vi "Close.vi"(7 "Micropulse # In":i32, 8 "error in (no error)":errorcluster) -> (0 "error out":errorcluster, 5 "Micropulse # Out":i32)   [LabVIEW 2026, in "MicroPulse_Driver.lvlib"]
doc: "Performs an instrument error query before terminating the software connection to the instrument."
uses:
  MicroPulse_Driver.lvlib
  Private/MP-Registry Action-Enum.ctl
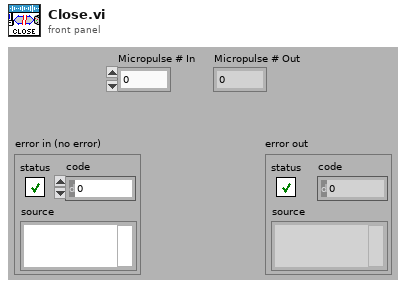
[diagram p1: front panel]
types:
  T1 = typedef "MicroPulse_Driver.lvlib/MP-Registry Action-Enum.ctl" = enum16{"Read", "Add Test", "Add Command", "Add Gate Command", "Add Encoder Command", "Clear Command  List", "Set Registry", "Set System Details", "Set DOF", "Set Velocity", "Disable Asynch Reads", "Enable Asynch Reads", "Add Connection", "Disconnect", "Shutdown"}
  T2 = typedef "MicroPulse_Driver.lvlib/TCP config.ctl" = cluster{"Connection ID":refnum<k5>, "IP address":string, "host port":u16, "OC timeout":i32, "Read timeout":i32, "Write timeout":i32}
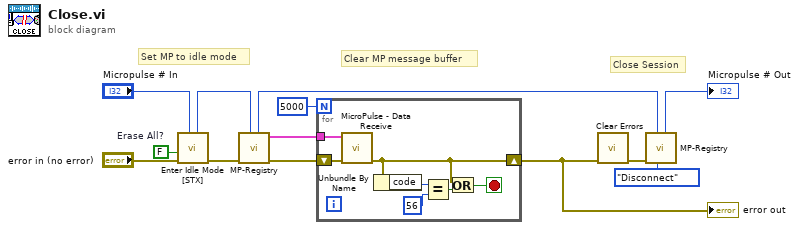
[diagram p0: block diagram]
diagram:
  w10 = FALSE  # Erase All?
  # "Set MP to idle mode"
  # "Clear MP message buffer"
  # "Close Session"
  n1 = call "Enter Idle Mode [STX].vi"("Micropulse # In"="Micropulse # In", "error in (no error)"="error in (no error)", "Erase All? (def T)"=w10) -> ("error out"=w6:errorcluster, "Micropulse # Out"=w2:i32)  [unwired: 7 in]
  n2 = call "MP-Registry.vi"("Micropulse # In"=w2, "error in (no error)"=w6) -> ("error out"=w5:errorcluster, "TCP config"=w4:T2, "Micropulse # Out"=w1:i32)  [unwired: 6 in, 1 out]
  n3 = for {
    N: 5000 -> [_]
    shift-right: [w14] -> w7
    shift-left: w5 -> [w19]
    tunnel: w4 -> [w20]
    stop <- w15 stop-if-true
    n4 = call "MicroPulse - Data Receive.vi"("error in (no error)"=w19, "TCP config"=w20) -> ("error out"=w14:errorcluster)  [unwired: 4 in, 5 out]
    n5 = Unbundle By Name(w14) -> ("code"=w18:i32)
    n6 = Equal?(x=w18, y=56) -> (x = y?=w16:bool)
    n7 = Or(x=w14, y=w16) -> (x .or. y?=w15:bool)
  }
  "error out" <- w7
  n8 = call <vilib>:"Clear Errors.vi"("error in (no error)"=w7) -> ("error out"=w9:errorcluster)  [unwired: 5 in, 1 out]
  n9 = call "MP-Registry.vi"("Action"=MP-Registry_Action-Enum."Disconnect", "Micropulse # In"=w1, "error in (no error)"=w9) -> ("Micropulse # Out"=→"Micropulse # Out":i32)  [unwired: 5 in, 3 out]
